vi "Array of Variants to Multi Dimensional Array Variant.vi"(7 "Dimension Lengths":i32[](array[numeric]), 8 "error in (no error)":errorcluster, 11 "[Variant]":variant[](array[variant])) -> (0 "error out":errorcluster, 3 "Array Variant":variant)   [LabVIEW 2018, in "TwinCAT ADS.lvclass"]
uses:
  TwinCAT ADS.lvclass
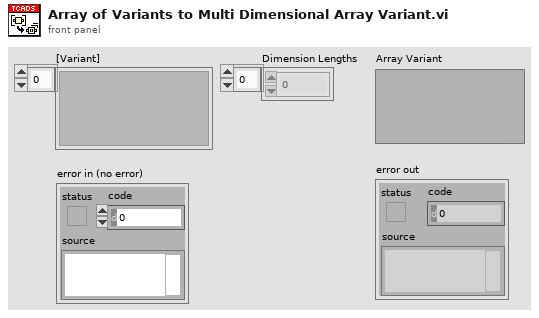
[diagram p1: front panel]
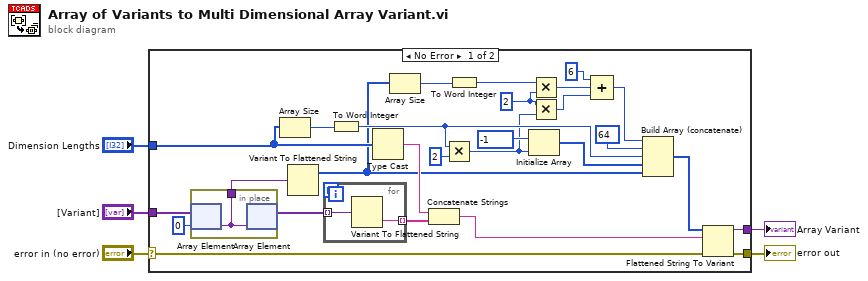
[diagram p0: block diagram]
diagram:
  n1 = case shown="No Error" "error in (no error)" {
    selector: "error in (no error)" -> [w30 w36]
    tunnel: [w29 w36] -> w4
    tunnel: "[Variant]" -> [w19 _]
    tunnel: [w28 _] -> w3
    tunnel: "Dimension Lengths" -> [w25 _]
    frame No Error {
      w9 = i16 2 ("y")
      n2 = in-place {
        in-place-border: [w33] -> w18
        n3 = in-place-array #1(w19, 0) -> (w33:variant)
        n4 = in-place-array #1(w33) -> (w16:variant[])  [unwired: 1 out]
      }
      n5 = Array Size(array=w25) -> (size(s)=w23:i32)
      n6 = Variant To Flattened String(Variant=w18) -> (1:w12:i16[])  [unwired: 1 out]
      n7 = for {
        tunnel: w16 -> [w35] mode=indexing
        tunnel: [w34] -> w20 mode=indexing
        n8 = Variant To Flattened String(Variant=w35) -> (data string=w34:string)  [unwired: 1 out]
      }
      n9 = To Word Integer(number=w23) -> (16bit integer=w22:i16)
      n10 = Type Cast(x=w25) -> (*(type *) &x=w32:string)  [unwired: 1 in]
      n11 = Array Size(array=w12) -> (size(s)=w11:i32)
      n12 = Concatenate Strings(w32, w20) -> (w24:string)
      n13 = Multiply(x=w22, y=i16 2) -> (x*y=w10:i16)
      n14 = To Word Integer(number=w11) -> (16bit integer=w7:i16)
      n15 = Initialize Array(i16 -1, w10) -> (w26:i16[])
      n16 = Multiply(x=w7, y=w9) -> (x*y=w13:i16)
      n17 = Multiply(x=w9, y=w10) -> (x*y=w8:i16)
      n18 = Compound Arithmetic op=ADD(i16 6 ("y"), w13, w8) -> (w14:i16)
      n19 = Build Array (concatenate)(w14, i16 64, w22, w26, w12) -> (w6:i16[])
      n20 = Flattened String To Variant(4:w30, 6:w24, 7:w6) -> (0:w29:errorcluster, 3:w28:variant)
    }
    frame Error {
    }
  }
  "error out" <- w4
  "Array Variant" <- w3
